vi "Tester.vi"() -> ()   [LabVIEW 2012]
uses:
  MB_PDU/MB_DevID Object.ctl
  <vilib>/NI/Modbus Library/Data Model/Device Data Model.lvclass
  <vilib>/NI/Modbus Library/API/Slave/Modbus Slave.lvclass
  <vilib>/NI/Modbus Library/API/Wrapper/Create TCP Slave.vi
  MB_Master_TCP.lvclass
  <vilib>/NI/Modbus Library/API/Wrapper/API Main.lvlib
  MB Master.lvlib
  MB_PDU/MB_ReadDevID Codes.ctl
panel:
  out "Conformity Level":u8
  out "DevID Objects":T1[](array[typedef])
  in  "stop server":bool
  out "error out":errorcluster
  in  "stop client":bool
  in  "Timeout (10000)":i32=1000
  in  "Port (502)":u16=502
  in  "IP Address":string="localhost"
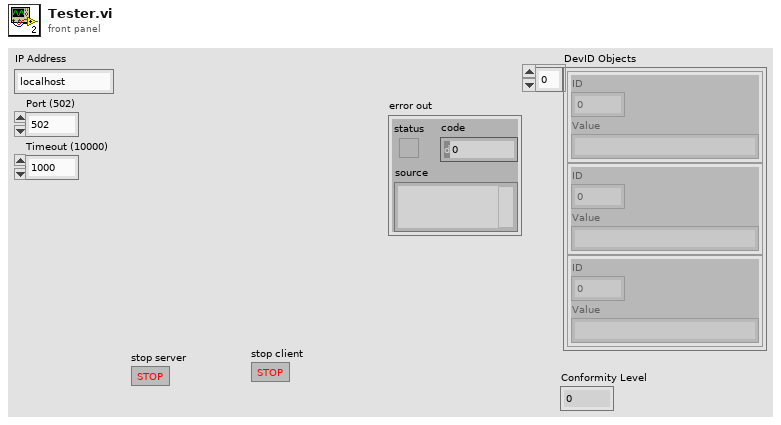
[diagram p1: front panel]
types:
  T1 = typedef "MB Master.lvlib/MB_DevID Object.ctl" = cluster{"ID":u8, "Value":string}
  T2 = typedef "MB Master.lvlib/MB_ReadDevID Codes.ctl" = u8
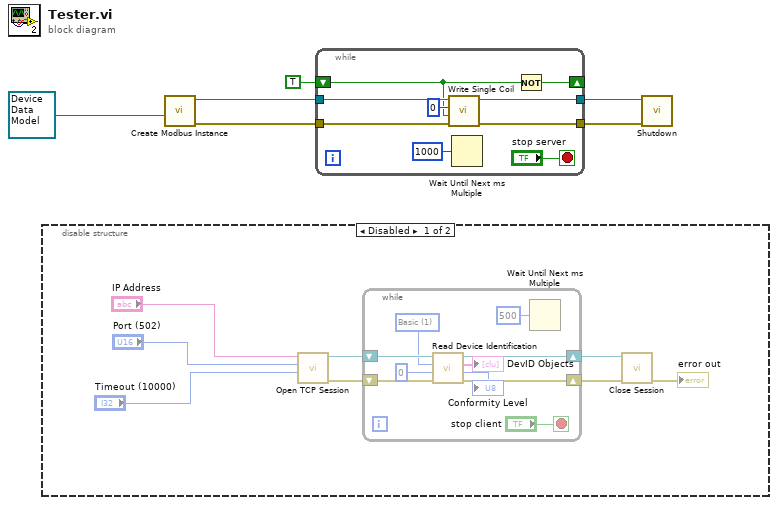
[diagram p0: block diagram]
diagram:
  n1 = disable-structure shown="Disabled" {
    frame Disabled {
      n2 = call "Open TCP Session.vi"("Timeout (10000)"="Timeout (10000)", "Port (502)"="Port (502)", "IP Address"="IP Address") -> ("error out"=w13:errorcluster, "MB_TCP session"=w14:refnum<class "MB_Master_TCP.lvclass">)  [unwired: 7 in]
      n3 = while {
        shift-right: [w19] -> w12
        shift-left: w14 -> [w22]
        shift-right: [w20] -> w11
        shift-left: w13 -> [w21]
        stop <- "stop client" stop-if-true
        w16 = T2 1 items=["Basic"=1, "Regular"=2, "Extended"=3, "Single"=4] ("read device ID code")
        n4 = call "Read Device Identification.vi"("error in (no error)"=w21, "object ID"=u8 0, "read device ID code"=w16, "MB session in"=w22) -> ("error out"=w20:errorcluster, "Conformity Level"=→"Conformity Level":u8, "DevID Objects"=→"DevID Objects":T1[], "MB session out"=w19:refnum<class "MB_Master_TCP.lvclass">)  [unwired: 4 in]
        n5 = Wait Until Next ms Multiple(millisecond multiple=u32 500) -> ()  [unwired: 1 out]
      }
      n6 = call-dynamic "Close Session.vi"("error in (no error)"=w11, "MB TCP session"=w12) -> ("error out"=→"error out":errorcluster)  [unwired: 9 in]
    }
    frame Enabled {
    }
  }
  n7 = call-poly <vilib>:"Create Modbus Instance.vi"("device data model"=refnum<class "Device Data Model.lvclass"> refnum) -> ("error out"=w4:errorcluster, "TCP slave instance"=w5:refnum<class "Modbus Slave.lvclass">)  [unwired: 9 in]
  n8 = while {
    tunnel: w5 -> [w33]
    tunnel: w4 -> [w31]
    tunnel: [w30] -> w3
    tunnel: [w29] -> w2
    shift-right: [w28] -> _
    shift-left: TRUE -> [w27]
    stop <- "stop server" stop-if-true
    n9 = call-dynamic "Write Single Coil.vi"("error in"=w31, "coil to write"=w27, "address"=u16 0, "Modbus slave in"=w33) -> ("error out"=w30:errorcluster, "Modbus slave out"=w29:refnum<class "Modbus Slave.lvclass">)  [unwired: 6 in]
    n10 = Wait Until Next ms Multiple(millisecond multiple=u32 1000) -> ()  [unwired: 1 out]
    n11 = Not(x=w27) -> (.not. x?=w28:bool)
  }
  n12 = call-dynamic "Shutdown.vi"("error in"=w3, "Modbus slave in"=w2) -> ()  [unwired: 9 in, 1 out]
